vi "Convert TDMS to XLSX.vi"(7 "replace?(T)":bool=TRUE, 8 "error in":errorcluster, 9 "Show Configure Dialog?":bool, 10 "Remove Extra Properties? (T)":bool=TRUE, 11 "Path to TDMS/TDM File":path) -> (0 "error out":errorcluster)   [LabVIEW 2018]
doc: "This VI will convert a TDMS file to a XLSX file. Excel 2007, and the TDMS Add on for Excel needs to be installed. Then provide the path to the TDMS or TDM file. A file with the same name in the same directory will be created with a .XLSX file extension.\n\nBy default the conversion will remove many extra properties that aren't always used. To include all properties make \"Remove Extra Properties\" false. If you would like to choose the properties to include set \"Show Configure Dialog\" to be true.\n\nBrian Hoover (hooovahh) 2010"
uses:
  <userlib>/_OpenG.lib/file/file.llb/Strip Path Extension - String__ogtk.vi
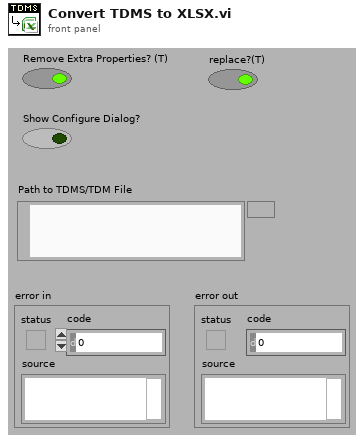
[diagram p1: front panel]
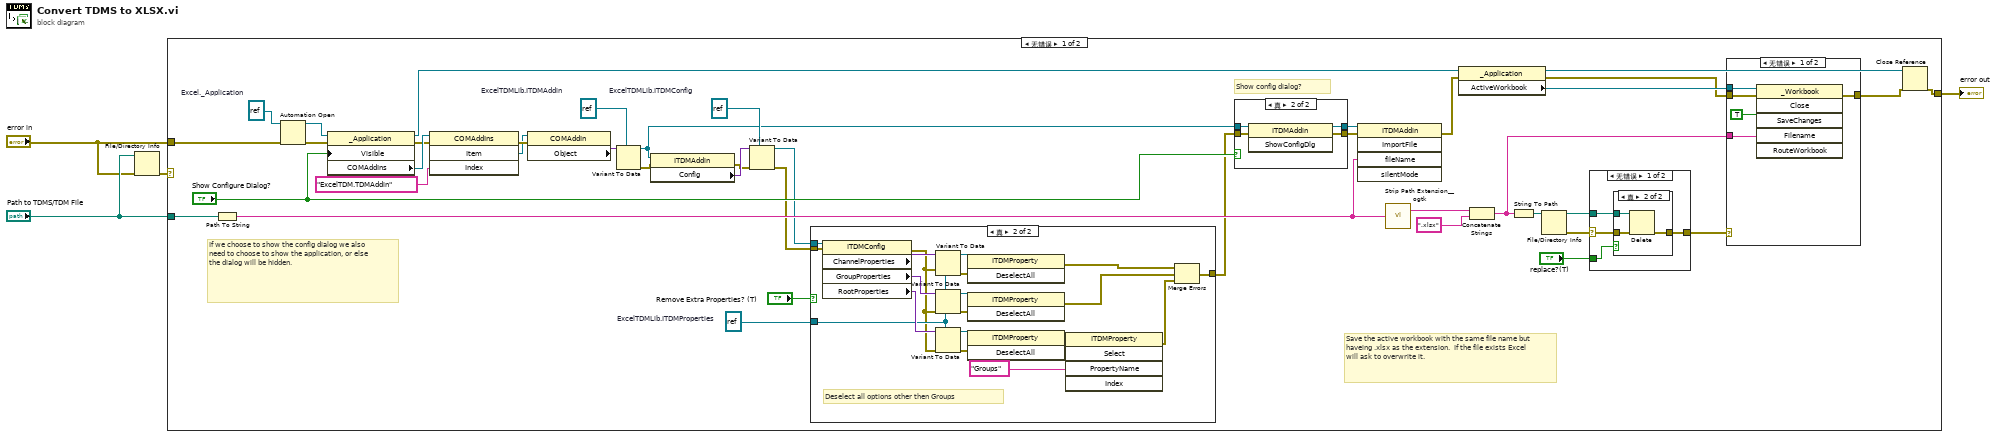
[diagram p0: block diagram]
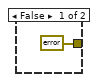
[diagram p2: hidden frame]
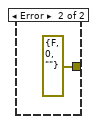
[diagram p3: hidden frame]
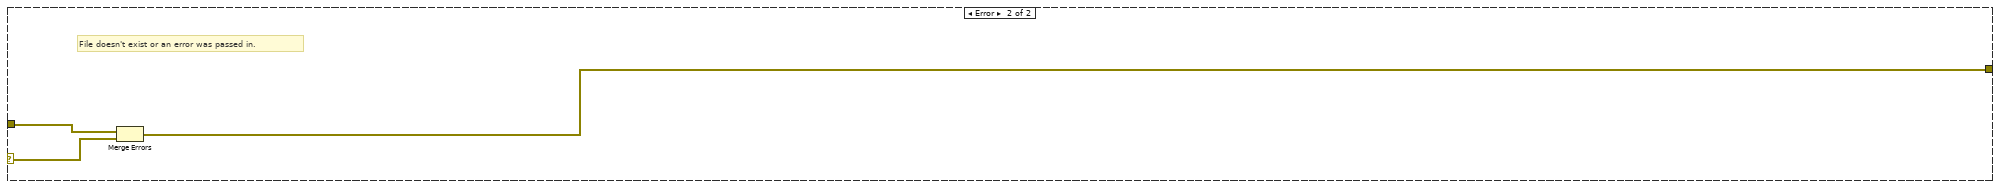
[diagram p7: hidden frame]
diagram:
  n1 = File/Directory Info(path="Path to TDMS/TDM File", error in="error in") -> (error out=w3:errorcluster)  [unwired: 6 out]
  n2 = case shown="无错误" w3 {
    selector: w3 -> [_ w89]
    tunnel: "Path to TDMS/TDM File" -> [w37 _]
    tunnel: [w14 w88] -> w1
    tunnel: "error in" -> [w32 w90]
    frame No Error {
      w11 = refnum<k7> refnum  # Excel._Application
      w26 = refnum<k7> refnum  # ExcelTDMLib.ITDMProperties
      w27 = refnum<k7> refnum  # ExcelTDMLib.ITDMConfig
      w44 = refnum<k7> refnum  # ExcelTDMLib.ITDMAddin
      # "Save the active workbook with the same file name but haveing .xlsx as the extension.  If the file exists Excel will ask to overwrite it."
      # "Show config dialog?"
      # "If we choose to show the config dialog we also need to choose to show the application, or else the dialog will be hidden."
      n3 = Path To String(path=w37) -> (string=w36:string)
      n4 = Automation Open(error in (no error)=w32, Automation Refnum=w11) -> (Automation Refnum=w6:refnum<k7>, error out=w43:errorcluster)  [unwired: 2 in]
      n5 = property class="_Application"(reference=w6, error in=w43, "Visible"="Show Configure Dialog?") -> (reference out=w16:refnum<k7>, error out=w40:errorcluster, "COMAddIns"=w45:refnum<k7>)
      n6 = invoke class="COMAddIns" method="Item"(reference=w45, error in=w40, "Index"="ExcelTDM.TDMAddin") -> (error out=w41:errorcluster, "Item"=w5:refnum<k7>)  [unwired: 1 in, 2 out]
      n7 = property class="COMAddIn"(reference=w5, error in=w41) -> ("Object"=w28:variant)  [unwired: 2 out]
      n8 = Variant To Data(type=w44, Variant=w28) -> (data=w25:refnum<k7>, error out=w23:errorcluster)  [unwired: 1 in]
      n9 = property class="ITDMAddin"(reference=w25, error in=w23) -> (error out=w22:errorcluster, "Config"=w24:variant)  [unwired: 1 out]
      n10 = Variant To Data(error in=w22, type=w27, Variant=w24) -> (data=w20:refnum<k7>, error out=w21:errorcluster)
      n11 = case shown="真" "Remove Extra Properties? (T)" {
        tunnel: w26 -> [_ w77]
        tunnel: w21 -> [w61 w68]
        tunnel: w20 -> [_ w67]
        tunnel: [w61 w66] -> w19
        frame False {
        }
        frame True {
          # "Deselect all options other then Groups"
          n12 = property class="ITDMConfig"(reference=w67, error in=w68) -> (error out=w72:errorcluster, "ChannelProperties"=w81:variant, "GroupProperties"=w79:variant, "RootProperties"=w78:variant)  [unwired: 1 out]
          n13 = Variant To Data(error in=w72, type=w77, Variant=w81) -> (data=w80:refnum<k7>, error out=w69:errorcluster)
          n14 = Variant To Data(error in=w72, type=w77, Variant=w79) -> (data=w75:refnum<k7>, error out=w70:errorcluster)
          n15 = Variant To Data(error in=w72, type=w77, Variant=w78) -> (data=w76:refnum<k7>, error out=w71:errorcluster)
          n16 = invoke class="ITDMProperty" method="DeselectAll"(reference=w80, error in=w69) -> (error out=w73:errorcluster)  [unwired: 1 in, 2 out]
          n17 = invoke class="ITDMProperty" method="DeselectAll"(reference=w75, error in=w70) -> (error out=w74:errorcluster)  [unwired: 1 in, 2 out]
          n18 = invoke class="ITDMProperty" method="DeselectAll"(reference=w76, error in=w71) -> (reference out=w65:refnum<k7>, error out=w64:errorcluster)  [unwired: 1 in, 1 out]
          n19 = invoke class="ITDMProperty" method="Select"(reference=w65, error in=w64, "PropertyName"="Groups" ("string")) -> (error out=w63:errorcluster)  [unwired: 2 in, 4 out]
          n20 = Merge Errors(w73, w74, w63) -> (w66:errorcluster)
        }
      }
      n21 = case shown="真" "Show Configure Dialog?" {
        tunnel: w25 -> [w83 w87]
        tunnel: w19 -> [w82 w86]
        tunnel: [w82 w85] -> w31
        tunnel: [w83 w84] -> w30
        frame False {
        }
        frame True {
          n22 = invoke class="ITDMAddin" method="ShowConfigDlg"(reference=w87, error in=w86) -> (reference out=w84:refnum<k7>, error out=w85:errorcluster)  [unwired: 1 in, 1 out]
        }
      }
      n23 = invoke class="ITDMAddin" method="ImportFile"(reference=w30, error in=w31, "fileName"=w36) -> (error out=w39:errorcluster)  [unwired: 2 in, 4 out]
      n24 = call-poly <userlib>:"Strip Path Extension__ogtk.vi"("path"=w36) -> ("root"=w35:string)  [unwired: 1 out]
      n25 = property class="_Application"(reference=w16, error in=w39) -> (reference out=w17:refnum<k7>, error out=w33:errorcluster, "ActiveWorkbook"=w38:refnum<k7>)
      n26 = Concatenate Strings(w35, ".xlsx" ("string")) -> (w13:string)
      n27 = String To Path(string=w13) -> (path=w12:path)
      n28 = File/Directory Info(path=w12) -> (path out=w8:path, error out=w10:errorcluster)  [unwired: 1 in, 5 out]
      n29 = case shown="无错误" w10 {
        selector: w10 -> [w47 _]
        tunnel: "replace?(T)" -> [w48 _]
        tunnel: w8 -> [w49 _]
        tunnel: [w46 errorcluster {"status"=FALSE, "code"=0, "source"=""} ("error out")] -> w7
        frame No Error {
          n30 = case shown="真" w48 {
            tunnel: w49 -> [_ w53]
            tunnel: w47 -> [_ w52]
            tunnel: [errorcluster {"status"=TRUE, "code"=0, "source"=""} ("error out") w51] -> w46
            frame False {
            }
            frame True {
              n31 = Delete(path (use dialog)=w53, error in=w52) -> (error out=w51:errorcluster)  [unwired: 3 in, 2 out]
            }
          }
        }
        frame Error {
        }
      }
      n32 = case shown="无错误" w7 {
        tunnel: w38 -> [w59 _]
        tunnel: w33 -> [w57 w60]
        tunnel: [w56 w60] -> w15
        tunnel: w13 -> [w55 _]
        frame No Error {
          n33 = invoke class="_Workbook" method="Close"(reference=w59, error in=w57, "SaveChanges"=TRUE, "Filename"=w55) -> (error out=w56:errorcluster)  [unwired: 2 in, 5 out]
        }
        frame Error {
        }
      }
      n34 = Close Reference(reference=w17, error in (no error)=w15) -> (error out=w14:errorcluster)
    }
    frame Error {
      # "File doesn't exist or an error was passed in."
      n35 = Merge Errors(w90, w89) -> (w88:errorcluster)
    }
  }
  "error out" <- w1
